vi "ISX3_Cmd_Reset.vi"() -> (0 "Reset Command":u8[](array[numeric]))   [LabVIEW 2012, in "Sciospec ISX3 Impedance Analyzer.lvlib"]
uses:
  Sciospec ISX3 Impedance Analyzer.lvlib
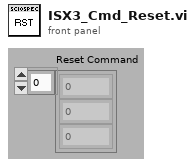
[diagram p1: front panel]
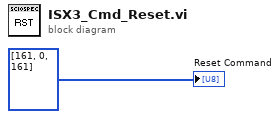
[diagram p0: block diagram]
diagram:
  "Reset Command" <- u8[] [161, 0, 161]
